vi "Auton_S1_Left_Scale.vi"   [LabVIEW 2017]
uses:
  <vilib>/Rock Robotics/WPI/Utilities/WPI_GetSetVariantRefNum.vi
  Robot Global Data.vi
  <vilib>/Rock Robotics/WPI/RobotDrive/WPI_RobotDriveArcadeDrive_Standard(NoSaturation).vi
types:
  T1 = typedef "WPI_RobotDriveDevRef.ctl" = cluster{"DevStatus":errorcluster, "Motors[]":T2[], "Square Inputs":bool, "Max Output":dbl}
  T2 = typedef "WPI_MotorControlDeviceRef.ctl" = cluster{"DeviceStatus":errorcluster, "Type":T3, "PWM":cluster{"PWM Channel":T4, "DeadBand":T5}, "CAN":cluster{"Device Number":u8, "SetOutput VI Ref":variant, "GetOutput VI Ref":variant, "Enable VI Ref":variant, "Disable VI Ref":variant, "Data":variant}, "Invert":bool, "DIO PWM":cluster{"PWM \"Enable\" Channel":T4, "DIOChannel":T6, "PWM Rate":dbl}}
  T3 = typedef "WPI_MotorControlType.ctl" = enum16{"PWM", "CAN", "DIO PWM"}
  T4 = typedef "FPGA_DIOPWMChannel.ctl" = enum8{"PWM 0", "PWM 1", "PWM 2", "PWM 3", "PWM 4", "PWM 5", "PWM 6", "PWM 7", "PWM 8", "PWM 9", "PWM MXP 0", "PWM MXP 1", "PWM MXP 2", "PWM MXP 3", "PWM MXP 4", "PWM MXP 5", "PWM MXP 6", "PWM MXP 7", "PWM MXP 8", "PWM MXP 9", "Invalid"}
  T5 = typedef "WPI_PWMDeadband.ctl" = cluster{"Name":string, "maxPositivePwm":i32, "minPositivePwm":i32, "centerPwm":i32, "maxNegativePwm":i32, "minNegativePwm":i32, "angularRange":u16}
  T6 = typedef "FPGA_DIOChannel.ctl" = enum8{"DIO 0", "DIO 1", "DIO 2", "DIO 3", "DIO 4", "DIO 5", "DIO 6", "DIO 7", "DIO 8", "DIO 9", "DIO MXP 0", "DIO MXP 1", "DIO MXP 2", "DIO MXP 3", "DIO MXP 4", "DIO MXP 5", "DIO MXP 6", "DIO MXP 7", "DIO MXP 8", "DIO MXP 9", "DIO MXP 10", "DIO MXP 11", "DIO MXP 12", "DIO MXP 13", "DIO MXP 14", "DIO MXP 15", "SPI Port CS1", "SPI Port CS2", "SPI Port CS3", "SPI Port MISO", "SPI Port MOSI", "Invalid"}
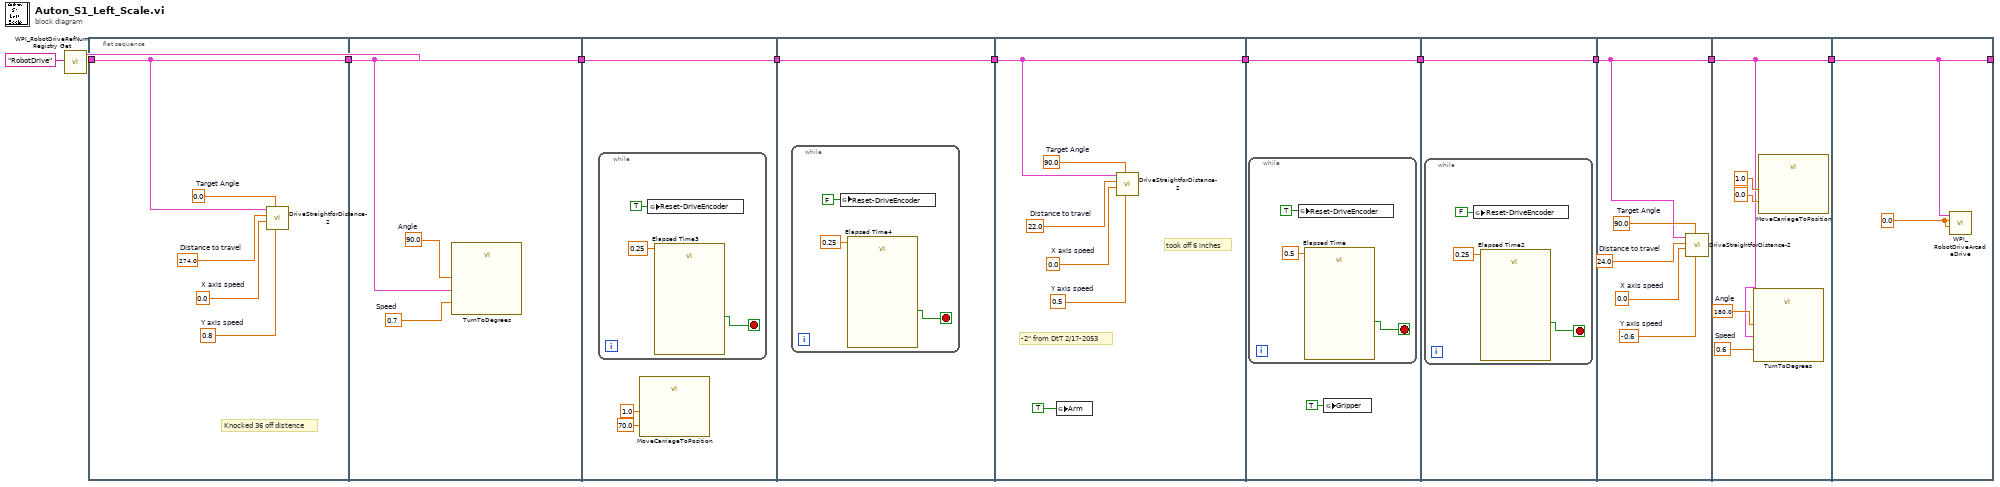
[diagram p0: block diagram]
diagram:
  n1 = call <vilib>:"WPI_RobotDriveRefNum Registry Get.vi"("refnum name"="RobotDrive") -> ("RobotDriveDevRef"=w7:T1)  [unwired: 9 in, 1 out]
  n2 = flat-sequence {
    tunnel: [w16] -> w11
    tunnel: w7 -> [w16]
    tunnel: w11 -> [w18]
    tunnel: [w18] -> w10
    tunnel: w10 -> [w22]
    tunnel: [w22] -> w9
    tunnel: [w26] -> w6
    tunnel: w9 -> [w26]
    tunnel: w6 -> [w31]
    tunnel: [w31] -> w5
    tunnel: w5 -> [w37]
    tunnel: [w37] -> w4
    tunnel: w4 -> [w41]
    tunnel: [w41] -> w3
    tunnel: w3 -> [w45]
    tunnel: [w45] -> w2
    tunnel: w2 -> [w50]
    tunnel: [w50] -> w1
    tunnel: [w55] -> _
    tunnel: w1 -> [w55]
    frame #0 {
      w12 = 0.0  # Target Angle
      w13 = 0.8  # Y axis speed
      w14 = 0.0  # X axis speed
      w15 = 274.0  # Distance to travel
      # "Knocked 36 off distence"
      n3 = call "DriveStraightforDistance-2.vi"("Y axis speed"=w13, "Target Angle"=w12, "X axis speed"=w14, "Distance to travel"=w15, "RobotDriveDevRef"=w16) -> ()  [unwired: 7 in]
    }
    frame #1 {
      w17 = 90.0  # Angle
      w19 = 0.7  # Speed
      n4 = call "TurnToDegrees.vi"("Speed"=w19, "RobotDriveDevRef"=w18, "Angle"=w17) -> ()  [unwired: 9 in]
    }
    frame #2 {
      n5 = while {
        stop <- w25 stop-if-true
        n6 = global write "Robot Global Data.vi" "Reset-DriveEncoder"(TRUE ("Reset-DriveEncoder")) -> ()
        n7 = call "Elapsed Time3"("Time Target (s)"=0.25) -> ("Time has Elapsed"=w25:bool)  [unwired: 11 in, 7 out]
      }
      n8 = call "MoveCarriageToPosition.vi"("Lift Speed"=1.0, "Target Height"=70.0) -> ()  [unwired: 10 in]
    }
    frame #3 {
      n9 = while {
        stop <- w29 stop-if-true
        n10 = global write "Robot Global Data.vi" "Reset-DriveEncoder"(FALSE ("Reset-DriveEncoder")) -> ()
        n11 = call "Elapsed Time4"("Time Target (s)"=0.25) -> ("Time has Elapsed"=w29:bool)  [unwired: 11 in, 7 out]
      }
    }
    frame #4 {
      w32 = 90.0  # Target Angle
      w33 = 0.5  # Y axis speed
      w34 = 0.0  # X axis speed
      w35 = 22.0  # Distance to travel
      # "took off 6 inches"
      # "-2\" from DtT 2/17-2053"
      n12 = global write "Robot Global Data.vi" "Arm"(TRUE ("Gripper")) -> ()
      n13 = call "DriveStraightforDistance-2.vi"("Y axis speed"=w33, "Target Angle"=w32, "X axis speed"=w34, "Distance to travel"=w35, "RobotDriveDevRef"=w31) -> ()  [unwired: 7 in]
    }
    frame #5 {
      n14 = while {
        stop <- w40 stop-if-true
        n15 = global write "Robot Global Data.vi" "Reset-DriveEncoder"(TRUE ("Reset-DriveEncoder")) -> ()
        n16 = call "Elapsed Time"("Time Target (s)"=0.5) -> ("Time has Elapsed"=w40:bool)  [unwired: 11 in, 7 out]
      }
      n17 = global write "Robot Global Data.vi" "Gripper"(TRUE ("Gripper")) -> ()
    }
    frame #6 {
      n18 = while {
        stop <- w44 stop-if-true
        n19 = global write "Robot Global Data.vi" "Reset-DriveEncoder"(FALSE ("Reset-DriveEncoder")) -> ()
        n20 = call "Elapsed Time2"("Time Target (s)"=0.25) -> ("Time has Elapsed"=w44:bool)  [unwired: 11 in, 7 out]
      }
    }
    frame #7 {
      w46 = 90.0  # Target Angle
      w47 = -0.6  # Y axis speed
      w48 = 0.0  # X axis speed
      w49 = 24.0  # Distance to travel
      n21 = call "DriveStraightforDistance-2.vi"("Y axis speed"=w47, "Target Angle"=w46, "X axis speed"=w48, "Distance to travel"=w49, "RobotDriveDevRef"=w45) -> ()  [unwired: 7 in]
    }
    frame #8 {
      w51 = 180.0  # Angle
      w52 = 0.6  # Speed
      n22 = call "TurnToDegrees.vi"("Speed"=w52, "RobotDriveDevRef"=w50, "Angle"=w51) -> ()  [unwired: 9 in]
      n23 = call "MoveCarriageToPosition.vi"("Lift Speed"=1.0, "Target Height"=0.0) -> ()  [unwired: 10 in]
    }
    frame #9 {
      w56 = 0.0 ("X axis value")
      n24 = call-poly <vilib>:"WPI_RobotDriveArcadeDrive.vi"("Y axis value"=w56, "X axis value"=w56, "RobotDriveDevRef"=w55) -> ()  [unwired: 6 in, 3 out]
    }
  }
